vi "Main.vi"   [LabVIEW 2019]
doc: "The myRIO Project template acquires acceleration data from the onboard accelerometer and displays the changes of acceleration values in a waveform chart."
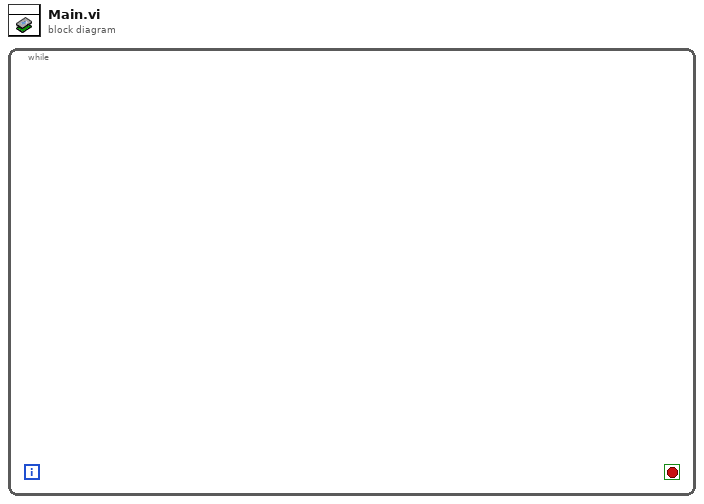
[diagram p0: block diagram]
diagram:
  n1 = while {
    stop <- _ stop-if-true
  }
